vi "Propriedades.vi"(4 "Cluster":T3, 5 "Propriedades":T2, 6 "Unidade":T1, 7 "Entry Type":T4, 8 "Fluid Name":T5) -> (3 "Valor Calculado":dbl)   [LabVIEW 2019]
uses:
  padrao_fluid_name_propriedades.ctl
  padrao_entry_type_propriedades.ctl
  padrao_propriedades_propriedades.ctl
  padrao_unidades_medida_propriedades.ctl
panel:
  out "Valor Propriedade 2":dbl
  out "Valor Propriedade 1":dbl
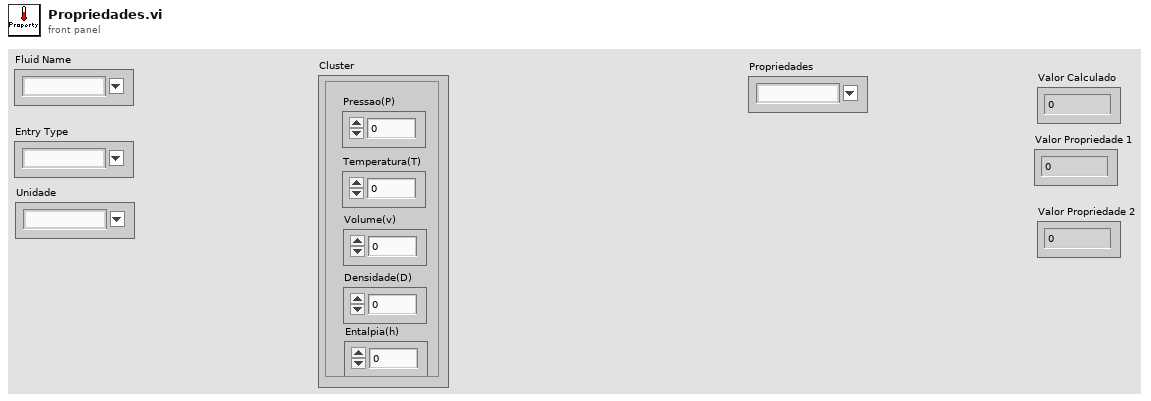
[diagram p1: front panel]
types:
  T1 = typedef "padrao_unidades_medida_propriedades.ctl" = string
  T2 = typedef "padrao_propriedades_propriedades.ctl" = string
  T3 = cluster{"Pressao(P)":dbl, "Temperatura(T)":dbl, "Volume(v)":dbl, "Densidade(D)":dbl, "Entalpia(h)":dbl}
  T4 = typedef "padrao_entry_type_propriedades.ctl" = string
  T5 = typedef "padrao_fluid_name_propriedades.ctl" = string
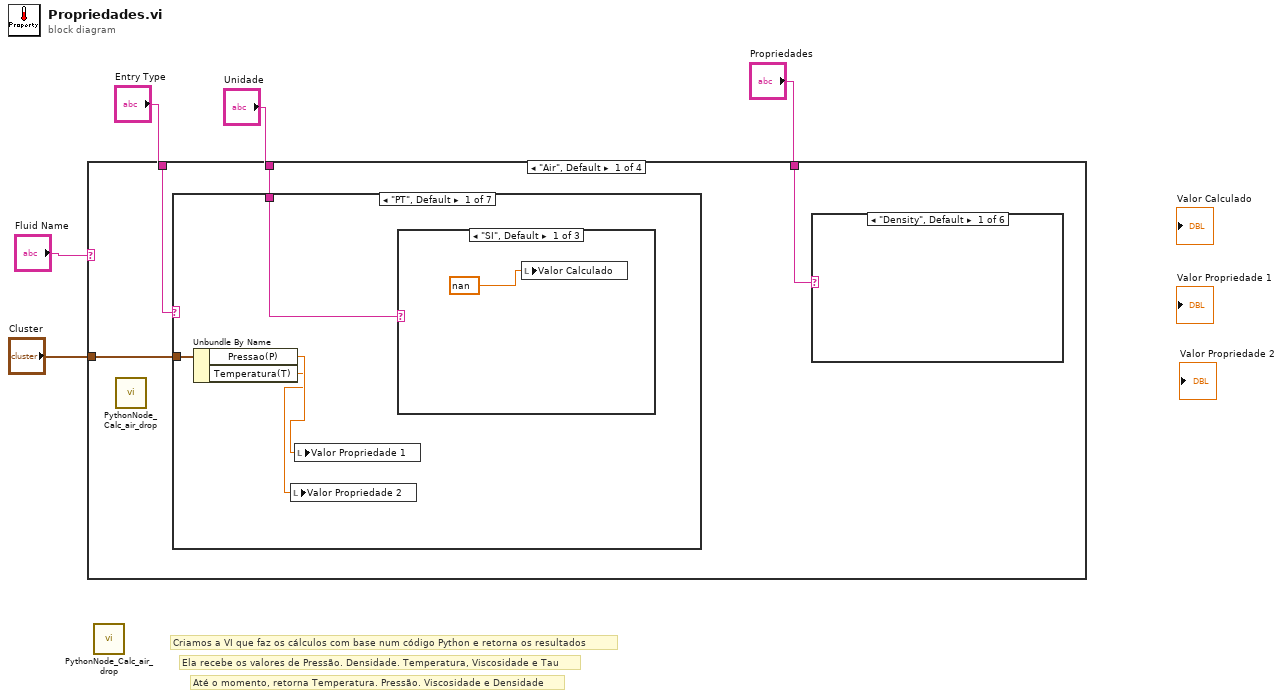
[diagram p0: block diagram]
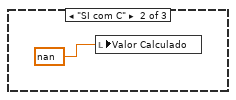
[diagram p7: hidden frame]
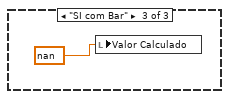
[diagram p8: hidden frame]
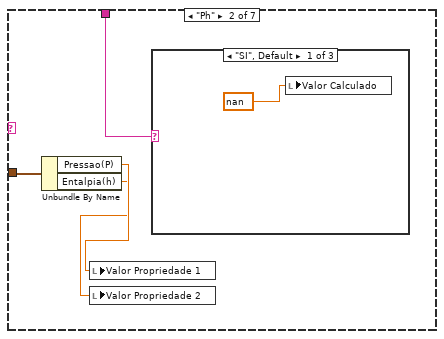
[diagram p9: hidden frame]
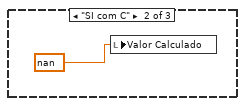
[diagram p10: hidden frame]
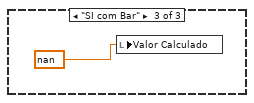
[diagram p11: hidden frame]
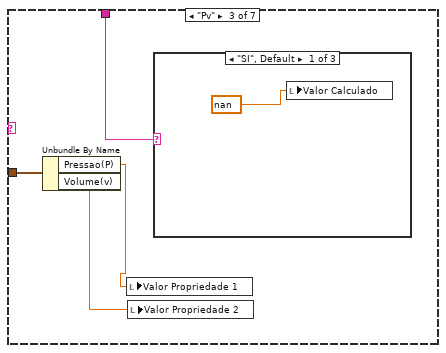
[diagram p12: hidden frame]
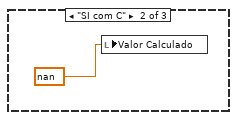
[diagram p13: hidden frame]
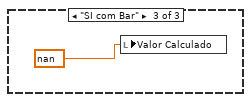
[diagram p14: hidden frame]
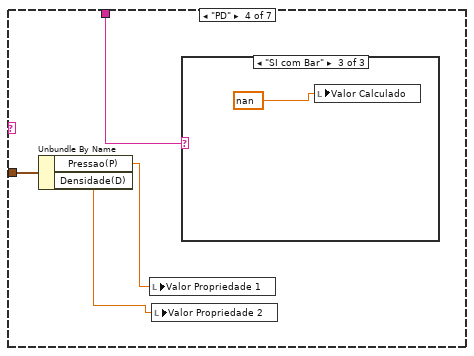
[diagram p15: hidden frame]
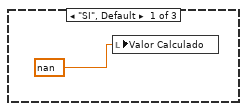
[diagram p16: hidden frame]
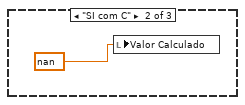
[diagram p17: hidden frame]
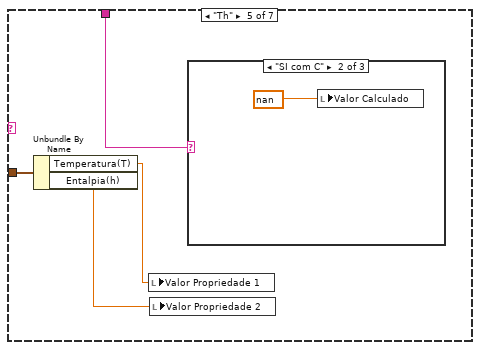
[diagram p18: hidden frame]
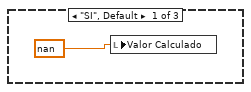
[diagram p19: hidden frame]
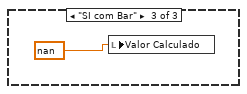
[diagram p20: hidden frame]
diagram:
  # "Até o momento, retorna Temperatura. Pressão. Viscosidade e Densidade"
  # "Ela recebe os valores de Pressão. Densidade. Temperatura, Viscosidade e Tau"
  # "Criamos a VI que faz os cálculos com base num código Python e retorna os resultados"
  n1 = case shown="\"Air\", Default" "Fluid Name" {
    tunnel: "Propriedades" -> [w9 w62 w91 w123]
    tunnel: "Unidade" -> [w8 w61 w94 w126]
    tunnel: "Entry Type" -> [w7 w60 w93 w125]
    tunnel: "Cluster" -> [w6 w59 w92 w124]
    frame "Air", Default {
      n2 = call "PythonNode_Calc_air_drop.vi"() -> ()  [unwired: 16 in]
      n3 = case shown="\"PT\", Default" w7 {
        tunnel: w8 -> [w13 w19 w26 w33 w40 w47 w54]
        tunnel: w6 -> [w12 w20 w27 w34 w41 w48 w55]
        frame "PT", Default {
          n4 = Unbundle By Name(w12) -> ("Pressao(P)"=w11:dbl, "Temperatura(T)"=w10:dbl)
          n5 = local write "Valor Propriedade 2"(w10) -> ()
          n6 = local write "Valor Propriedade 1"(w11) -> ()
          n7 = case shown="\"SI\", Default" w13 {
            frame "SI", Default {
              n8 = local write "Valor Calculado"(nan) -> ()
            }
            frame "SI com C" {
              n9 = local write "Valor Calculado"(nan) -> ()
            }
            frame "SI com Bar" {
              n10 = local write "Valor Calculado"(nan) -> ()
            }
          }
        }
        frame "Ph" {
          n11 = Unbundle By Name(w20) -> ("Pressao(P)"=w18:dbl, "Entalpia(h)"=w17:dbl)
          n12 = local write "Valor Propriedade 1"(w18) -> ()
          n13 = local write "Valor Propriedade 2"(w17) -> ()
          n14 = case shown="\"SI\", Default" w19 {
            frame "SI", Default {
              n15 = local write "Valor Calculado"(nan) -> ()
            }
            frame "SI com C" {
              n16 = local write "Valor Calculado"(nan) -> ()
            }
            frame "SI com Bar" {
              n17 = local write "Valor Calculado"(nan) -> ()
            }
          }
        }
        frame "Pv" {
          n18 = Unbundle By Name(w27) -> ("Pressao(P)"=w25:dbl, "Volume(v)"=w24:dbl)
          n19 = local write "Valor Propriedade 1"(w25) -> ()
          n20 = local write "Valor Propriedade 2"(w24) -> ()
          n21 = case shown="\"SI\", Default" w26 {
            frame "SI", Default {
              n22 = local write "Valor Calculado"(nan) -> ()
            }
            frame "SI com C" {
              n23 = local write "Valor Calculado"(nan) -> ()
            }
            frame "SI com Bar" {
              n24 = local write "Valor Calculado"(nan) -> ()
            }
          }
        }
        frame "PD" {
          n25 = Unbundle By Name(w34) -> ("Pressao(P)"=w32:dbl, "Densidade(D)"=w31:dbl)
          n26 = local write "Valor Propriedade 1"(w32) -> ()
          n27 = local write "Valor Propriedade 2"(w31) -> ()
          n28 = case shown="\"SI com Bar\"" w33 {
            frame "SI", Default {
              n29 = local write "Valor Calculado"(nan) -> ()
            }
            frame "SI com C" {
              n30 = local write "Valor Calculado"(nan) -> ()
            }
            frame "SI com Bar" {
              n31 = local write "Valor Calculado"(nan) -> ()
            }
          }
        }
        frame "Th" {
          n32 = Unbundle By Name(w41) -> ("Temperatura(T)"=w39:dbl, "Entalpia(h)"=w38:dbl)
          n33 = local write "Valor Propriedade 1"(w39) -> ()
          n34 = local write "Valor Propriedade 2"(w38) -> ()
          n35 = case shown="\"SI com C\"" w40 {
            frame "SI", Default {
              n36 = local write "Valor Calculado"(nan) -> ()
            }
            frame "SI com C" {
              n37 = local write "Valor Calculado"(nan) -> ()
            }
            frame "SI com Bar" {
              n38 = local write "Valor Calculado"(nan) -> ()
            }
          }
        }
        frame "Tv" {
          n39 = Unbundle By Name(w48) -> ("Temperatura(T)"=w46:dbl, "Volume(v)"=w45:dbl)
          n40 = case shown="\"SI com C\"" w47 {
            frame "SI", Default {
              n41 = local write "Valor Calculado"(nan) -> ()
            }
            frame "SI com C" {
              n42 = local write "Valor Calculado"(nan) -> ()
            }
            frame "SI com Bar" {
              n43 = local write "Valor Calculado"(nan) -> ()
            }
          }
          n44 = local write "Valor Propriedade 1"(w46) -> ()
          n45 = local write "Valor Propriedade 2"(w45) -> ()
        }
        frame "TD" {
          n46 = Unbundle By Name(w55) -> ("Temperatura(T)"=w53:dbl, "Densidade(D)"=w52:dbl)
          n47 = local write "Valor Propriedade 1"(w53) -> ()
          n48 = local write "Valor Propriedade 2"(w52) -> ()
          n49 = case shown="\"SI\", Default" w54 {
            frame "SI", Default {
              n50 = local write "Valor Calculado"(nan) -> ()
            }
            frame "SI com C" {
              n51 = local write "Valor Calculado"(nan) -> ()
            }
            frame "SI com Bar" {
              n52 = local write "Valor Calculado"(nan) -> ()
            }
          }
        }
      }
      n53 = case shown="\"Density\", Default" w9 {
        frame "Density", Default {
        }
        frame "Volume" {
        }
        frame "Pressure" {
        }
        frame "Temperature" {
        }
        frame "Viscosity" {
        }
        frame "Entalpia" {
        }
      }
    }
    frame "Water" {
      n54 = call "PythonNode_Calc_air_drop.vi"() -> ()  [unwired: 16 in]
      n55 = case shown="\"Tv\"" w60 {
        tunnel: w61 -> [w65 w69 w74 w77 w81 w86 w89]
        tunnel: w59 -> [w66 w70 w73 w78 w82 w85 w90]
        frame "PT", Default {
          n56 = Unbundle By Name(w66) -> ("Pressao(P)"=w64:dbl, "Temperatura(T)"=w63:dbl)
          n57 = case shown="\"SI\", Default" w65 {
            frame "SI", Default {
            }
            frame "SI com C" {
            }
            frame "SI com Bar" {
            }
          }
          n58 = local write "Valor Propriedade 1"(w64) -> ()
          n59 = local write "Valor Propriedade 2"(w63) -> ()
        }
        frame "Ph" {
          n60 = Unbundle By Name(w70) -> ("Pressao(P)"=w68:dbl, "Entalpia(h)"=w67:dbl)
          n61 = local write "Valor Propriedade 1"(w68) -> ()
          n62 = local write "Valor Propriedade 2"(w67) -> ()
          n63 = case shown="\"SI\", Default" w69 {
            frame "SI", Default {
            }
            frame "SI com C" {
            }
            frame "SI com Bar" {
            }
          }
        }
        frame "Pv" {
          n64 = Unbundle By Name(w73) -> ("Pressao(P)"=w72:dbl, "Volume(v)"=w71:dbl)
          n65 = case shown="\"SI com Bar\"" w74 {
            frame "SI", Default {
            }
            frame "SI com C" {
            }
            frame "SI com Bar" {
            }
          }
          n66 = local write "Valor Propriedade 1"(w72) -> ()
          n67 = local write "Valor Propriedade 2"(w71) -> ()
        }
        frame "PD" {
          n68 = Unbundle By Name(w78) -> ("Pressao(P)"=w76:dbl, "Densidade(D)"=w75:dbl)
          n69 = local write "Valor Propriedade 1"(w76) -> ()
          n70 = local write "Valor Propriedade 2"(w75) -> ()
          n71 = case shown="\"SI\", Default" w77 {
            frame "SI", Default {
            }
            frame "SI com C" {
            }
            frame "SI com Bar" {
            }
          }
        }
        frame "Th" {
          n72 = Unbundle By Name(w82) -> ("Temperatura(T)"=w80:dbl, "Entalpia(h)"=w79:dbl)
          n73 = local write "Valor Propriedade 1"(w80) -> ()
          n74 = local write "Valor Propriedade 2"(w79) -> ()
          n75 = case shown="\"SI\", Default" w81 {
            frame "SI", Default {
            }
            frame "SI com C" {
            }
            frame "SI com Bar" {
            }
          }
        }
        frame "Tv" {
          n76 = Unbundle By Name(w85) -> ("Temperatura(T)"=w84:dbl, "Volume(v)"=w83:dbl)
          n77 = local write "Valor Propriedade 1"(w84) -> ()
          n78 = local write "Valor Propriedade 2"(w83) -> ()
          n79 = case shown="\"SI\", Default" w86 {
            frame "SI", Default {
            }
            frame "SI com C" {
            }
            frame "SI com Bar" {
            }
          }
        }
        frame "TD" {
          n80 = Unbundle By Name(w90) -> ("Temperatura(T)"=w88:dbl, "Densidade(D)"=w87:dbl)
          n81 = local write "Valor Propriedade 1"(w88) -> ()
          n82 = local write "Valor Propriedade 2"(w87) -> ()
          n83 = case shown="\"SI com C\"" w89 {
            frame "SI", Default {
            }
            frame "SI com C" {
            }
            frame "SI com Bar" {
            }
          }
        }
      }
      n84 = case shown="\"Entalpia\"" w62 {
        frame "Density", Default {
        }
        frame "Volume" {
        }
        frame "Pressure" {
        }
        frame "Temperature" {
        }
        frame "Viscosity" {
        }
        frame "Entalpia" {
        }
      }
    }
    frame "Kerosene" {
      n85 = call "PythonNode_Calc_air_drop.vi"() -> ()  [unwired: 16 in]
      n86 = case shown="\"Pv\"" w93 {
        tunnel: w94 -> [w98 w102 w106 w110 w114 w118 w122]
        tunnel: w92 -> [w97 w101 w105 w109 w113 w117 w121]
        frame "PT", Default {
          n87 = Unbundle By Name(w97) -> ("Pressao(P)"=w96:dbl, "Temperatura(T)"=w95:dbl)
          n88 = local write "Valor Propriedade 1"(w96) -> ()
          n89 = local write "Valor Propriedade 2"(w95) -> ()
          n90 = case shown="\"SI\", Default" w98 {
            frame "SI", Default {
            }
            frame "SI com C" {
            }
            frame "SI com Bar" {
            }
          }
        }
        frame "Ph" {
          n91 = Unbundle By Name(w101) -> ("Pressao(P)"=w100:dbl, "Entalpia(h)"=w99:dbl)
          n92 = local write "Valor Propriedade 1"(w100) -> ()
          n93 = local write "Valor Propriedade 2"(w99) -> ()
          n94 = case shown="\"SI\", Default" w102 {
            frame "SI", Default {
            }
            frame "SI com C" {
            }
            frame "SI com Bar" {
            }
          }
        }
        frame "Pv" {
          n95 = Unbundle By Name(w105) -> ("Pressao(P)"=w104:dbl, "Volume(v)"=w103:dbl)
          n96 = local write "Valor Propriedade 1"(w104) -> ()
          n97 = local write "Valor Propriedade 2"(w103) -> ()
          n98 = case shown="\"SI com Bar\"" w106 {
            frame "SI", Default {
            }
            frame "SI com C" {
            }
            frame "SI com Bar" {
            }
          }
        }
        frame "PD" {
          n99 = Unbundle By Name(w109) -> ("Pressao(P)"=w108:dbl, "Densidade(D)"=w107:dbl)
          n100 = local write "Valor Propriedade 1"(w108) -> ()
          n101 = local write "Valor Propriedade 2"(w107) -> ()
          n102 = case shown="\"SI\", Default" w110 {
            frame "SI", Default {
            }
            frame "SI com C" {
            }
            frame "SI com Bar" {
            }
          }
        }
        frame "Th" {
          n103 = Unbundle By Name(w113) -> ("Temperatura(T)"=w112:dbl, "Entalpia(h)"=w111:dbl)
          n104 = local write "Valor Propriedade 1"(w112) -> ()
          n105 = local write "Valor Propriedade 2"(w111) -> ()
          n106 = case shown="\"SI\", Default" w114 {
            frame "SI", Default {
            }
            frame "SI com C" {
            }
            frame "SI com Bar" {
            }
          }
        }
        frame "Tv" {
          n107 = Unbundle By Name(w117) -> ("Temperatura(T)"=w116:dbl, "Volume(v)"=w115:dbl)
          n108 = local write "Valor Propriedade 1"(w116) -> ()
          n109 = local write "Valor Propriedade 2"(w115) -> ()
          n110 = case shown="\"SI\", Default" w118 {
            frame "SI", Default {
            }
            frame "SI com C" {
            }
            frame "SI com Bar" {
            }
          }
        }
        frame "TD" {
          n111 = Unbundle By Name(w121) -> ("Temperatura(T)"=w120:dbl, "Densidade(D)"=w119:dbl)
          n112 = local write "Valor Propriedade 1"(w120) -> ()
          n113 = local write "Valor Propriedade 2"(w119) -> ()
          n114 = case shown="\"SI\", Default" w122 {
            frame "SI", Default {
            }
            frame "SI com C" {
            }
            frame "SI com Bar" {
            }
          }
        }
      }
      n115 = case shown="\"Entalpia\"" w91 {
        frame "Density", Default {
        }
        frame "Volume" {
        }
        frame "Pressure" {
        }
        frame "Temperature" {
        }
        frame "Viscosity" {
        }
        frame "Entalpia" {
        }
      }
    }
    frame "R410A" {
      n116 = call "PythonNode_Calc_air_drop.vi"() -> ()  [unwired: 16 in]
      n117 = case shown="\"PT\", Default" w125 {
        tunnel: w126 -> [w130 w134 w138 w142 w146 w153 w157]
        tunnel: w124 -> [w129 w133 w137 w141 w145 w152 w156]
        frame "PT", Default {
          n118 = Unbundle By Name(w129) -> ("Pressao(P)"=w128:dbl, "Temperatura(T)"=w127:dbl)
          n119 = local write "Valor Propriedade 1"(w128) -> ()
          n120 = local write "Valor Propriedade 2"(w127) -> ()
          n121 = case shown="\"SI\", Default" w130 {
            frame "SI", Default {
            }
            frame "SI com C" {
            }
            frame "SI com Bar" {
            }
          }
        }
        frame "Ph" {
          n122 = Unbundle By Name(w133) -> ("Pressao(P)"=w132:dbl, "Entalpia(h)"=w131:dbl)
          n123 = case shown="\"SI\", Default" w134 {
            frame "SI", Default {
            }
            frame "SI com C" {
            }
            frame "SI com Bar" {
            }
          }
          n124 = local write "Valor Propriedade 1"(w132) -> ()
          n125 = local write "Valor Propriedade 2"(w131) -> ()
        }
        frame "Pv" {
          n126 = Unbundle By Name(w137) -> ("Pressao(P)"=w136:dbl, "Volume(v)"=w135:dbl)
          n127 = case shown="\"SI com Bar\"" w138 {
            frame "SI", Default {
            }
            frame "SI com C" {
            }
            frame "SI com Bar" {
            }
          }
          n128 = local write "Valor Propriedade 1"(w136) -> ()
          n129 = local write "Valor Propriedade 2"(w135) -> ()
        }
        frame "PD" {
          n130 = Unbundle By Name(w141) -> ("Pressao(P)"=w140:dbl, "Densidade(D)"=w139:dbl)
          n131 = local write "Valor Propriedade 1"(w140) -> ()
          n132 = local write "Valor Propriedade 2"(w139) -> ()
          n133 = case shown="\"SI\", Default" w142 {
            frame "SI", Default {
            }
            frame "SI com C" {
            }
            frame "SI com Bar" {
            }
          }
        }
        frame "Th" {
          n134 = Unbundle By Name(w145) -> ("Temperatura(T)"=w144:dbl, "Entalpia(h)"=w143:dbl)
          n135 = local write "Valor Propriedade 1"(w144) -> ()
          n136 = local write "Valor Propriedade 2"(w143) -> ()
          n137 = case shown="\"SI\", Default" w146 {
            frame "SI", Default {
              n138 = local write "Valor Calculado"(nan) -> ()
            }
            frame "SI com C" {
              n139 = local write "Valor Calculado"(nan) -> ()
            }
            frame "SI com Bar" {
              n140 = local write "Valor Calculado"(nan) -> ()
            }
          }
        }
        frame "Tv" {
          n141 = Unbundle By Name(w152) -> ("Temperatura(T)"=w151:dbl, "Volume(v)"=w150:dbl)
          n142 = local write "Valor Propriedade 1"(w151) -> ()
          n143 = local write "Valor Propriedade 2"(w150) -> ()
          n144 = case shown="\"SI\", Default" w153 {
            frame "SI", Default {
            }
            frame "SI com C" {
            }
            frame "SI com Bar" {
            }
          }
        }
        frame "TD" {
          n145 = Unbundle By Name(w156) -> ("Temperatura(T)"=w155:dbl, "Densidade(D)"=w154:dbl)
          n146 = local write "Valor Propriedade 1"(w155) -> ()
          n147 = local write "Valor Propriedade 2"(w154) -> ()
          n148 = case shown="\"SI\", Default" w157 {
            frame "SI", Default {
            }
            frame "SI com C" {
            }
            frame "SI com Bar" {
            }
          }
        }
      }
      n149 = case shown="\"Density\", Default" w123 {
        frame "Density", Default {
        }
        frame "Volume" {
        }
        frame "Pressure" {
        }
        frame "Temperature" {
        }
        frame "Viscosity" {
        }
        frame "Entalpia" {
        }
      }
    }
  }
  n150 = call "PythonNode_Calc_air_drop.vi"() -> ()  [unwired: 16 in]
